vi "read text file.vi"(8 "error in":errorcluster, 11 "file path in":path) -> (0 "error out":errorcluster, 2 "text":string, 3 "path out":path)   [LabVIEW 2023, in "Reusable Library.lvlib"]
uses:
  Reusable Library.lvlib
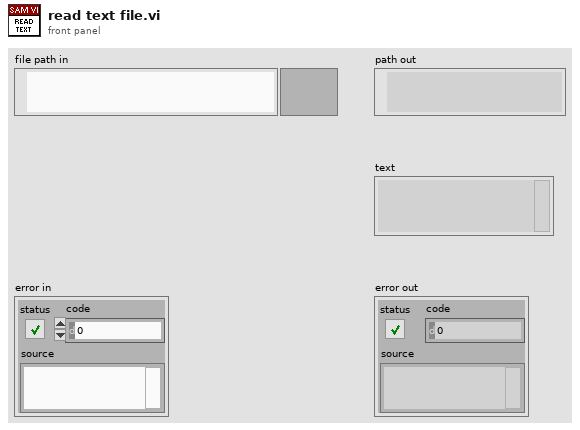
[diagram p1: front panel]
types:
  T1 = enum16{"open", "replace", "create", "open or create", "replace or create", "replace or create with confirmation"}
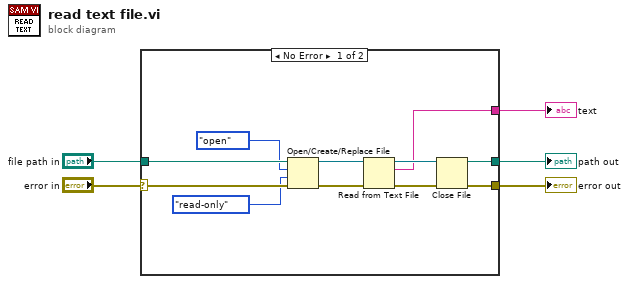
[diagram p0: block diagram]
diagram:
  n1 = case shown="No Error" "error in" {
    selector: "error in" -> [w9 w17]
    tunnel: [w6 _] -> w5
    tunnel: "file path in" -> [w12 w18]
    tunnel: [w11 w18] -> w3
    tunnel: [w10 w17] -> w2
    frame No Error {
      n2 = Open/Create/Replace File(file path (use dialog)=w12, error in=w9, operation (0:open)=T1."open", access (0:read/write)=enum16{"read/write", "read-only", "write-only"}."read-only") -> (refnum out=w16:refnum<file>, error out=w14:errorcluster)  [unwired: 2 in, 1 out]
      n3 = Read from Text File(file (use dialog)=w16, error in=w14) -> (refnum out=w15:refnum<file>, text=w6:string, error out=w13:errorcluster)  [unwired: 2 in, 1 out]
      n4 = Close File(refnum=w15, error in=w13) -> (path=w11:path, error out=w10:errorcluster)
    }
    frame Error {
    }
  }
  "text" <- w5
  "path out" <- w3
  "error out" <- w2
